vi "ATS_Binary_File_Write.vi"(9 "Data_In":u16[](array[numeric]), 10 "Write_Ctrl":enum16{"Open", "Write", "Close"}(ring)) -> (0 "error out":errorcluster, 3 "new file path":path)   [LabVIEW 2012]
doc: "Shows a quick way to write a binary byte stream file to disk with simple error checking. Run the Read Binary File example to read the file."
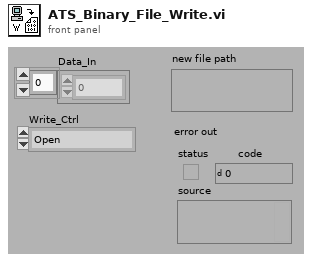
[diagram p1: front panel]
types:
  T1 = enum16{"open", "open or create", "create or replace", "create", "open (read only)"}
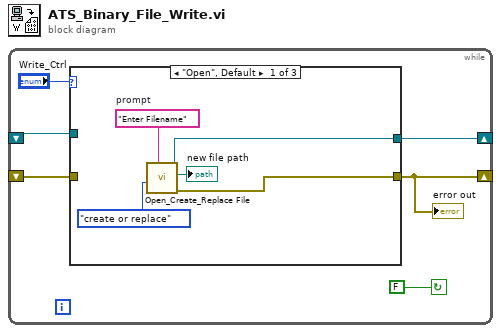
[diagram p0: block diagram]
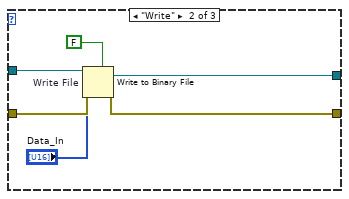
[diagram p2: hidden frame]
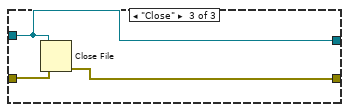
[diagram p3: hidden frame]
diagram:
  n1 = while {
    shift-right: [w4] -> _
    shift-left: _ -> [w1]
    shift-right: [w3] -> _
    shift-left: _ -> [w2]
    stop <- FALSE continue-if-true
    n2 = case shown="\"Open\", Default" "Write_Ctrl" {
      tunnel: [w9 w13 w20] -> w4
      tunnel: [w8 w14 w19] -> w3
      tunnel: w2 -> [_ w17 w18]
      tunnel: w1 -> [_ w15 w20]
      frame "Open", Default {
        w11 = "Enter Filename"  # prompt
        n3 = call <vilib>:"Open_Create_Replace File.vi"("prompt"=w11, "function (open:0)"=T1."create or replace") -> ("error out"=w8:errorcluster, "new file path"=→"new file path":path, "refnum"=w9:refnum<file>)  [unwired: 6 in, 1 out]
      }
      frame "Write" {
        n4 = Write to Binary File "Write File"(file (use dialog)=w15, data="Data_In", error in=w17, 5:FALSE ("prepend array or string size? (T)")) -> (refnum out=w13:refnum<file>, error out=w14:errorcluster)  [unwired: 2 in, 1 out]
      }
      frame "Close" {
        n5 = Close File(refnum=w20, error in=w18) -> (error out=w19:errorcluster)  [unwired: 1 out]
      }
    }
    "error out" <- w3
  }
